vi "Replace_Array_Subset.vi"(0 "Element RAS":i8=-10, 1 "Subarray RAS":i8[](array[numeric])=[-5, -8], 2 "Index RAS":i32, 3 "RAS1D":i8[](array[numeric])=[100, -1, -2, 9, 10], 4 "Indexs RAS":T1={"Rows"=-1, "Columns"=-1} {"Columns" min=-1; "Rows" min=-1}, 5 "RAS2D":i8[][](array[numeric])=[[0, 4, 7], [0, 5, 8], [3, 6, 9]], 6 "E or S RAS":T2, 8 "Choose RAS":T3) -> (15 "New Array RAS1D":i8[](array[numeric]), 18 "New Array RAS2D":i8[][](array[numeric]))   [LabVIEW 2018]
uses:
  Controls/1D_2D.ctl
  Controls/E_S.ctl
  Controls/Rows_Columns.ctl
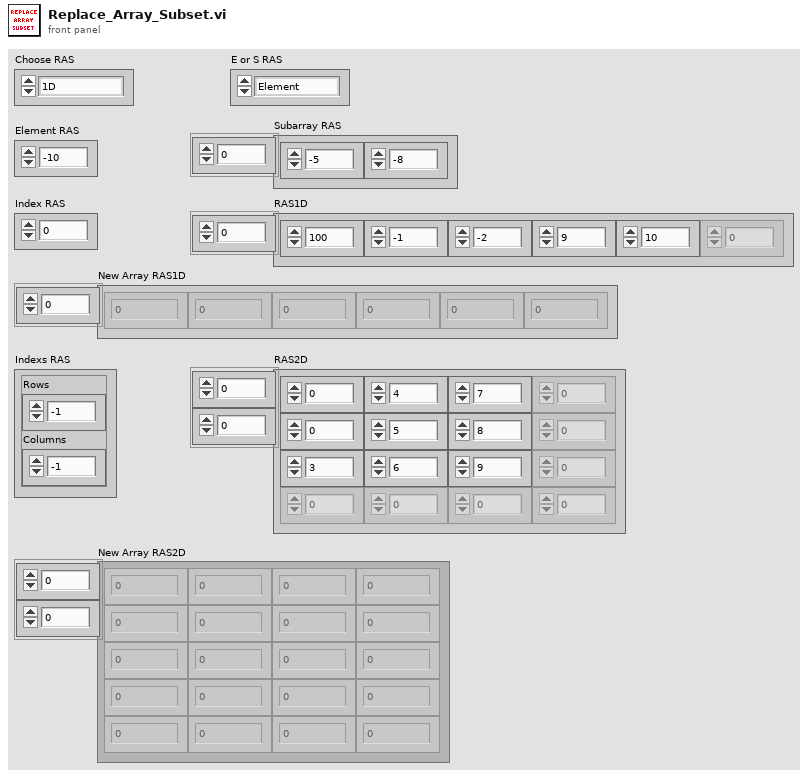
[diagram p1: front panel]
types:
  T1 = typedef "Rows_Columns.ctl" = cluster{"Rows":i32, "Columns":i32}
  T2 = typedef "E_S.ctl" = enum16{"Element", "SubArray"}
  T3 = typedef "1D_2D.ctl" = enum16{"1D", "2D"}
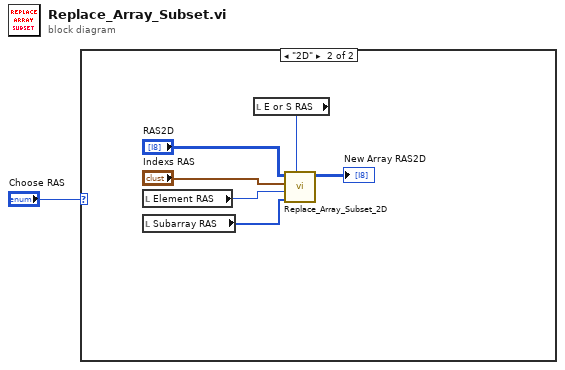
[diagram p0: block diagram]
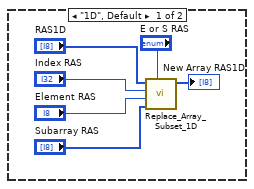
[diagram p2: hidden frame]
diagram:
  n1 = case shown="\"2D\"" "Choose RAS" {
    frame "1D", Default {
      n2 = call "Replace_Array_Subset_1D.vi"("E or S RAS"="E or S RAS", "Subarray RAS"="Subarray RAS", "Element RAS"="Element RAS", "Index RAS"="Index RAS", "RAS1D"="RAS1D") -> ("New Array RAS1D"=→"New Array RAS1D":i8[])  [unwired: 6 in]
    }
    frame "2D" {
      n3 = local read "Element RAS"() -> (w9:i8)
      n4 = local read "Subarray RAS"() -> (w8:i8[])
      n5 = local read "E or S RAS"() -> (w13:T2)
      n6 = call "Replace_Array_Subset_2D.vi"("E or S RAS"=w13, "SubArray RAS"=w8, "Element RAS"=w9, "Indexs RAS"="Indexs RAS", "RAS2D"="RAS2D") -> ("New Array RAS2D"=→"New Array RAS2D":i8[][])  [unwired: 6 in]
    }
  }
